vi "Call.vi"(7 "LabVIEW Web Service Request":refnum<class "Web Request.lvclass">) -> ()   [LabVIEW 2015]
uses:
  <vilib>/wsapi/Web Request.lvclass
  Classes/Server/Send Request (Sync).vi
  Classes/Server/JSONRPC Server.lvclass
panel:
  # "Use the Web Service Request input terminal to call the VIs on the Web Services palette. Do not remove it from the connector pane unless you don't need access to the palette."
  # "Each additional control wired to the connector pane will be available as an input in the URL. To include an indicator in terminal-mode output (the default setting), it must also be wired to the connector pane."
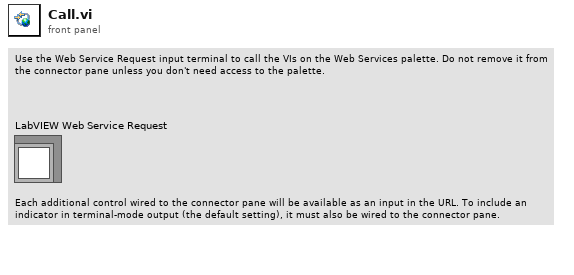
[diagram p1: front panel]
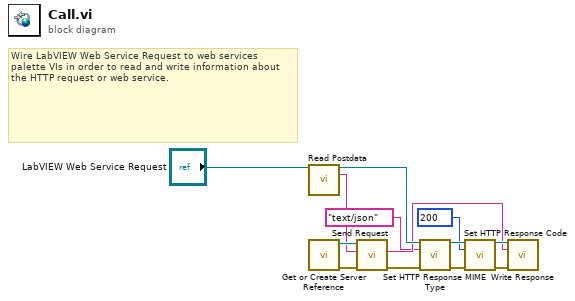
[diagram p0: block diagram]
diagram:
  w6 = 200 items=["100"=100, "101"=101, "200"=200, "201"=201, "202"=202, "203"=203, "204"=204, "205"=205, "206"=206, "300"=300, "301"=301, "302"=302, "303"=303, "304"=304, "305"=305, "306"=306, "307"=307, "400"=400, "401"=401, "402"=402, "403"=403, "404"=404, "405"=405, "406"=406, "407"=407, "408"=408, "409"=409, "410"=410, "411"=411, "412"=412, "413"=413, "414"=414, "415"=415, "416"=416, "417"=417, "500"=500, "501"=501, "502"=502, "503"=503, "504"=504, "505"=505] ("response code (200)")
  # "Wire LabVIEW Web Service Request to web services palette VIs in order to read and write information about the HTTP request or web service."
  n1 = call <vilib>:"Read Postdata.vi"("LabVIEW Web Service Request"="LabVIEW Web Service Request") -> ("LabVIEW Web Service Request out"=w5:refnum<class "Web Request.lvclass">, "postdata"=w11:string)  [unwired: 12 in, 1 out]
  n2 = call "Get or Create Server Reference.vi"() -> ("error out"=w2:errorcluster, "Server Out"=w12:refnum<class "JSONRPC Server.lvclass">)  [unwired: 10 in]
  n3 = call-poly "Send Request.vi"("error in (no error)"=w2, "JSON Request String"=w11, "JSONRPC Server in"=w12) -> ("error out"=w1:errorcluster, "JSON Response String"=w4:string)  [unwired: 6 in, 1 out]
  n4 = call <vilib>:"Set HTTP Response MIME Type.vi"("LabVIEW Web Service Request"=w5, "MIME type (text/html)"="text/json", "error in (no error)"=w1) -> ("LabVIEW Web Service Request out"=w8:refnum<class "Web Request.lvclass">, "error out"=w7:errorcluster)  [unwired: 11 in]
  n5 = call <vilib>:"Set HTTP Response Code.vi"("LabVIEW Web Service Request"=w8, "response code (200)"=w6, "error in (no error)"=w7) -> ("LabVIEW Web Service Request out"=w10:refnum<class "Web Request.lvclass">, "error out"=w9:errorcluster)  [unwired: 11 in]
  n6 = call <vilib>:"Write Response.vi"("LabVIEW Web Service Request"=w10, "response string"=w4, "error in (no error)"=w9) -> ()  [unwired: 11 in, 2 out]
